vi "DigitalFilter.vi"(7 "Filter":T1, 9 "FilterParams":variant, 10 "Original Data":dbl[](array[numeric])) -> (2 "Output":dbl[](array[numeric]))   [LabVIEW 2013]
uses:
  ControlDef/ProcessingMode.ctl
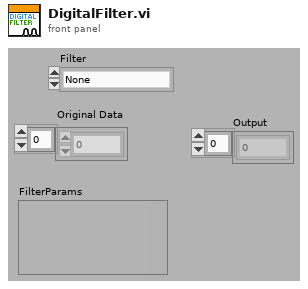
[diagram p1: front panel]
types:
  T1 = typedef "ProcessingMode.ctl" = enum16{"None", "Drop by Threshold", "TDC Simulate", "SetFilter"}
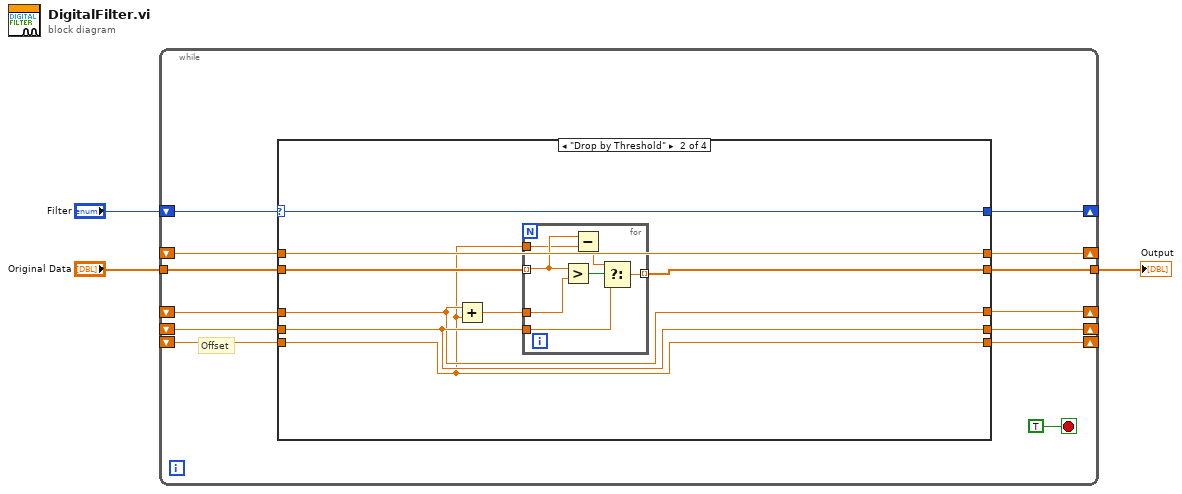
[diagram p0: block diagram]
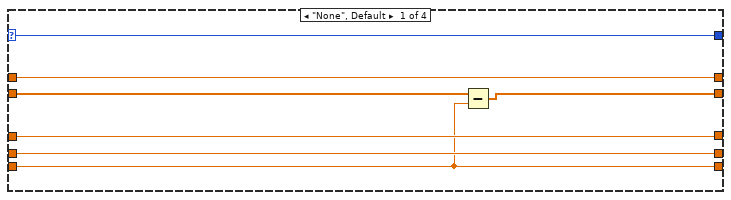
[diagram p2: hidden frame]
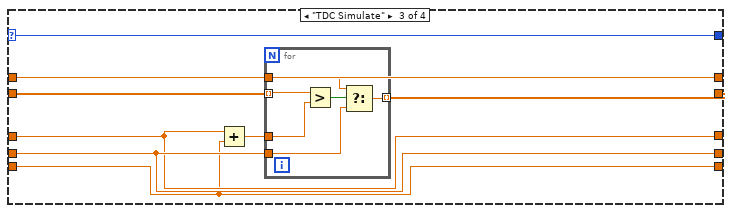
[diagram p3: hidden frame]
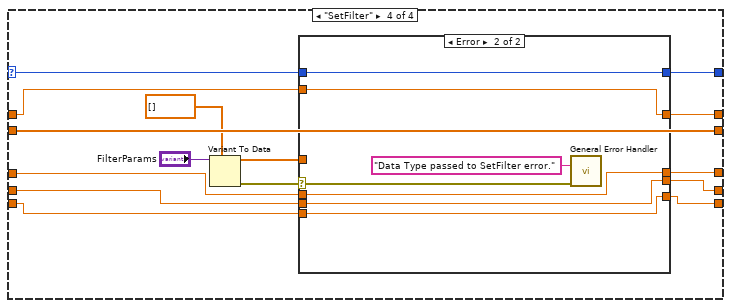
[diagram p4: hidden frame]
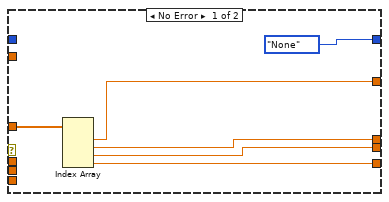
[diagram p5: hidden frame]
diagram:
  n1 = while {
    tunnel: [w14] -> w3
    tunnel: "Original Data" -> [w13]
    shift-right: [w10] -> _
    shift-left: _ -> [w16]
    shift-right: [w8] -> _
    shift-left: _ -> [w11]
    shift-right: [w9] -> _
    shift-left: _ -> [w15]
    shift-right: [w6] -> _
    shift-left: _ -> [w5]
    shift-right: [w4] -> _
    shift-left: "Filter" -> [w12]
    stop <- TRUE stop-if-true
    # "Offset"
    n2 = case shown="\"Drop by Threshold\"" w12 {
      selector: w12 -> [w17 w27 w42 w57]
      tunnel: w16 -> [w21 w26 w41 w55]
      tunnel: w15 -> [w20 w31 w46 w54]
      tunnel: [w19 w30 w44 w67] -> w14
      tunnel: w13 -> [w23 w29 w45 w67]
      tunnel: w11 -> [w22 w28 w43 w56]
      tunnel: [w21 w26 w41 w64] -> w10
      tunnel: [w20 w31 w46 w63] -> w9
      tunnel: [w22 w28 w43 w62] -> w8
      tunnel: [w18 w24 w39 w59] -> w6
      tunnel: w5 -> [w18 w24 w39 w53]
      tunnel: [w17 w27 w42 w58] -> w4
      frame "None", Default {
        n3 = Subtract(x=w23, y=w18) -> (x-y=w19:dbl[])
      }
      frame "Drop by Threshold" {
        n4 = Add(x=w26, y=w24) -> (x+y=w25:dbl)
        n5 = for {
          tunnel: w29 -> [w37] mode=indexing
          tunnel: [w36] -> w30 mode=indexing
          tunnel: w31 -> [w35]
          tunnel: w25 -> [w34]
          tunnel: w24 -> [w32]
          n6 = Greater?(x=w37, y=w34) -> (0:w38:bool)
          n7 = Subtract(x=w37, y=w32) -> (x-y=w33:dbl)
          n8 = Select(t=w33, s=w38, f=w35) -> (s? t:f=w36:dbl)
        }
      }
      frame "TDC Simulate" {
        n9 = Add(x=w41, y=w39) -> (x+y=w40:dbl)
        n10 = for {
          tunnel: w45 -> [w51] mode=indexing
          tunnel: [w50] -> w44 mode=indexing
          tunnel: w46 -> [w49]
          tunnel: w40 -> [w48]
          tunnel: w43 -> [w47]
          n11 = Greater?(x=w51, y=w48) -> (0:w52:bool)
          n12 = Select(t=w47, s=w52, f=w49) -> (s? t:f=w50:dbl)
        }
      }
      frame "SetFilter" {
        n13 = Variant To Data(type=dbl[] [], Variant="FilterParams") -> (data=w65:dbl[], error out=w60:errorcluster)  [unwired: 1 in]
        n14 = case shown="Error" w60 {
          selector: w60 -> [_ w75]
          tunnel: w65 -> [w73 _]
          tunnel: [w71 w78] -> w64
          tunnel: [w70 w77] -> w63
          tunnel: [w72 w79] -> w62
          tunnel: [w69 w76] -> w59
          tunnel: [ProcessingMode."None" ("Filter") w80] -> w58
          tunnel: w57 -> [_ w80]
          tunnel: w56 -> [_ w79]
          tunnel: w55 -> [_ w78]
          tunnel: w54 -> [_ w77]
          tunnel: w53 -> [_ w76]
          frame No Error {
            n15 = Index Array(array=w73) -> (element #1=w72:dbl, element #2=w71:dbl, element #3=w70:dbl, element #4=w69:dbl)  [unwired: 4 in]
          }
          frame Error {
            n16 = call <vilib>:"General Error Handler.vi"("[error source] (\" \")"="Data Type passed to SetFilter error." ("[error source] (\" \")"), "error in (no error)"=w75) -> ()  [unwired: 9 in, 5 out]
          }
        }
      }
    }
  }
  "Output" <- w3
